vi "CLK机柜开关切换.vi"(6 "OUT":u16, 7 "IN":u16, 8 "error in":errorcluster caption="error constant", 11 "CLK":refnum<k5>) -> (0 "error out":errorcluster caption="error constant", 2 "ask":string)   [LabVIEW 2015]
uses:
  server/Global/SeverGlobal.vi
panel:
  out "Isfailed":bool
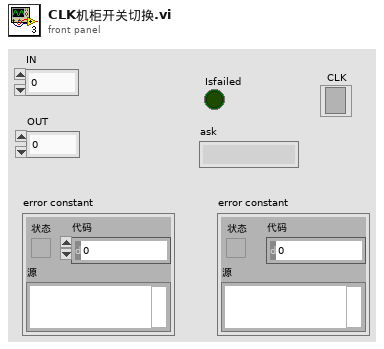
[diagram p1: front panel]
types:
  T1 = enum16{"Standard", "Buffered", "CRLF", "Immediate"}
  T2 = cluster{"IP_A":string, "PORT_A":i32, "IP_B":string, "PORT_B":i32, "IP_CLK":string, "PORT_CLK":i32, "IP_SWITCH":string, "PORT_SWITCH":i32}
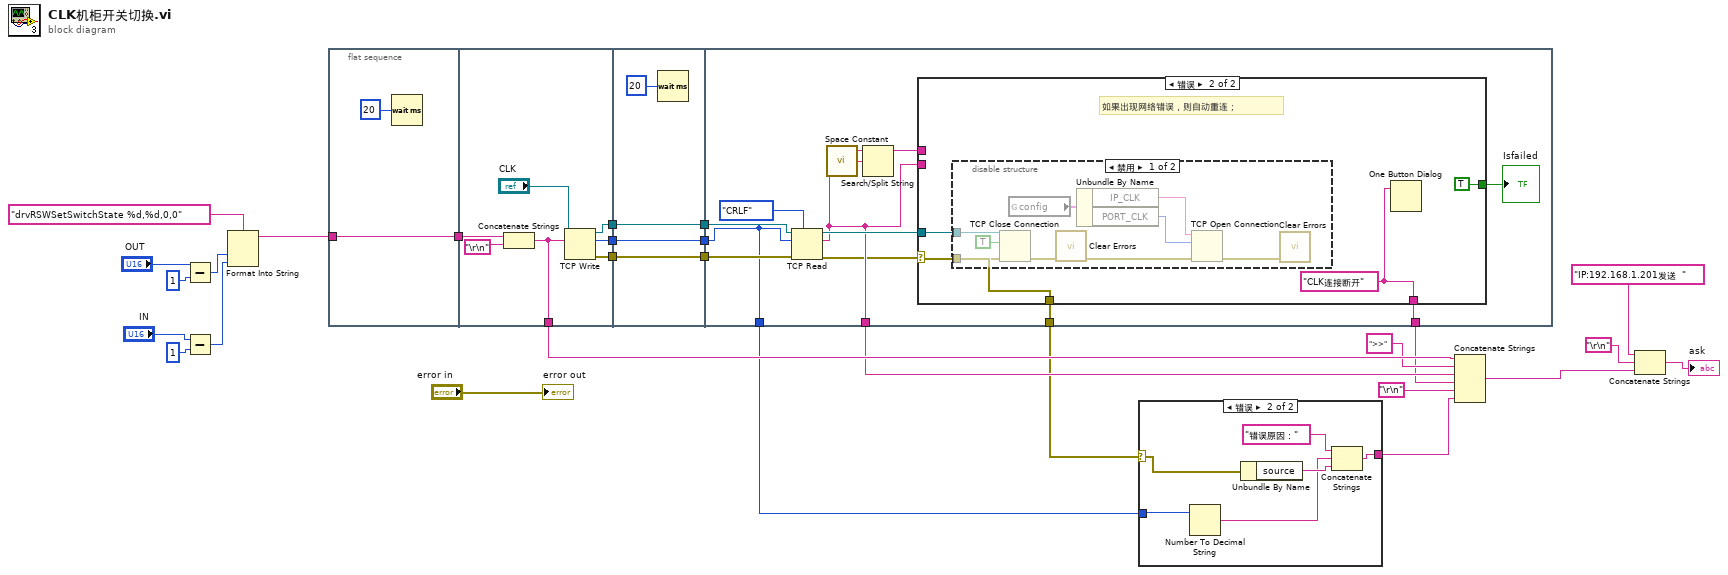
[diagram p0: block diagram]
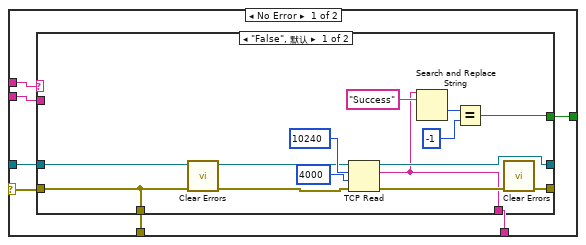
[diagram p3: hidden frame]
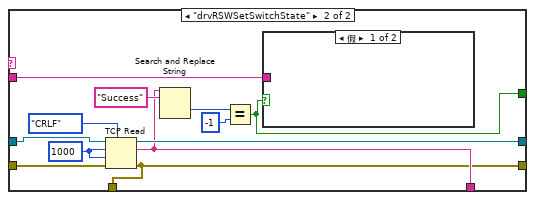
[diagram p4: hidden frame]
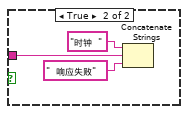
[diagram p5: hidden frame]
diagram:
  n1 = Subtract(x="OUT", y=1) -> (x-y=w19:i32)
  n2 = Subtract(x="IN", y=1) -> (x-y=w17:i32)
  n3 = Format Into String(format string="drvRSWSetSwitchState %d,%d,0,0" ("格式字符串"), w19, w17) -> (resulting string=w16:string)  [unwired: 2 in, 1 out]
  n4 = flat-sequence {
    tunnel: w16 -> [w30]
    tunnel: [w30] -> w28
    tunnel: [w35] -> w27
    tunnel: [w34] -> w26
    tunnel: [w33] -> w25
    tunnel: [w32] -> w9
    tunnel: w28 -> [w36]
    tunnel: [w40] -> w24
    tunnel: w27 -> [w40]
    tunnel: [w39] -> w23
    tunnel: w26 -> [w39]
    tunnel: [w38] -> w22
    tunnel: w25 -> [w38]
    tunnel: w24 -> [w49]
    tunnel: w23 -> [w42]
    tunnel: w22 -> [w48]
    tunnel: [w46] -> w7
    tunnel: [w45] -> w6
    tunnel: [w44] -> w4
    tunnel: [w42] -> w1
    frame #0 {
      n5 = Wait (ms)(milliseconds to wait=u32 20 ("delay")) -> ()  [unwired: 1 out]
    }
    frame #1 {
      n6 = Concatenate Strings(w36, "\r\n") -> (w32:string)
      n7 = TCP Write(connection ID="CLK", data in=w32) -> (connection ID out=w35:refnum<k5>, bytes written=w34:i32, error out=w33:errorcluster)  [unwired: 2 in]
    }
    frame #2 {
      n8 = Wait (ms)(milliseconds to wait=u32 20 ("delay")) -> ()  [unwired: 1 out]
    }
    frame #3 {
      n9 = TCP Read(connection ID=w49, bytes to read=w42, error in (no error)=w48, 7:T1."CRLF" ("mode (standard)")) -> (connection ID out=w50:refnum<k5>, data out=w46:string, error out=w43:errorcluster)  [unwired: 1 in]
      n10 = call <vilib>:"Space Constant.vi"() -> ("String"=w53:string)
      n11 = Search/Split String(string=w46, search string/char (-)=w53) -> (substring before match=w51:string)  [unwired: 1 in, 2 out]
      n12 = case shown="错误" w43 {
        selector: w43 -> [w54 w90]
        tunnel: w51 -> [w60 _]
        tunnel: w50 -> [w59 w92]
        tunnel: [w58 TRUE] -> w47
        tunnel: w46 -> [w57 _]
        tunnel: [w56 w89] -> w45
        tunnel: [w55 w90] -> w44
        frame No Error {
          n13 = case shown="\"False\", 默认" w60 {
            tunnel: [w69 w84] -> _
            tunnel: [w68 w74] -> _
            tunnel: w59 -> [w70 w83]
            tunnel: w54 -> [w61 w82]
            tunnel: w57 -> [_ w77]
            tunnel: [w63 w76] -> w58
            tunnel: [w64 w75] -> w56
            tunnel: [w61 w74] -> w55
            frame "False", Default {
              n14 = call <vilib>:"Clear Errors.vi"("error in (no error)"=w61) -> ("error out"=w62:errorcluster)  [unwired: 5 in, 1 out]
              n15 = TCP Read(connection ID=w70, bytes to read=10240, error in (no error)=w62, 9:4000 ("timeout ms (25000)")) -> (connection ID out=w69:refnum<k5>, data out=w64:string, error out=w72:errorcluster)  [unwired: 1 in]
              n16 = Search and Replace String(input string=w64, search string="Success") -> (offset past replacement=w65:i32)  [unwired: 6 in, 3 out]
              n17 = Equal?(x=w65, y=-1) -> (x = y?=w63:bool)
              n18 = call <vilib>:"Clear Errors.vi"("error in (no error)"=w72) -> ("error out"=w68:errorcluster)  [unwired: 5 in, 1 out]
            }
            frame "drvRSWSetSwitchState" {
              w81 = 1000 ("timeout ms (25000)")
              n19 = TCP Read(connection ID=w83, bytes to read=w81, error in (no error)=w82, 7:T1."CRLF" ("mode (standard)"), 9:w81) -> (connection ID out=w84:refnum<k5>, data out=w75:string, error out=w74:errorcluster)
              n20 = Search and Replace String(input string=w75, search string="Success") -> (offset past replacement=w79:i32)  [unwired: 6 in, 3 out]
              n21 = Equal?(x=w79, y=-1) -> (x = y?=w76:bool)
              n22 = case shown="假" w76 {
                tunnel: w77 -> [_ w88]
                frame False {
                }
                frame True {
                  n23 = Concatenate Strings("时钟  " ("message"), w88, "  响应失败" ("message")) -> ()  [unwired: 1 out]
                }
              }
            }
          }
        }
        frame Error {
          w89 = "CLK连接断开" ("字符串")
          # "如果出现网络错误，则自动重连；"
          n24 = disable-structure shown="禁用" {
            disable-tunnel: w92 -> [w95 _]
            disable-tunnel: w90 -> [w94 _]
            frame Disabled {
              n25 = TCP Close Connection(connection ID=w95, abort (F)=TRUE ("中止(F)"), error in (no error)=w94) -> (error out=w96:errorcluster)  [unwired: 1 out]
              n26 = global read "SeverGlobal.vi" "config"() -> (w98:T2)
              n27 = call <vilib>:"Clear Errors.vi"("error in (no error)"=w96) -> ("error out"=w97:errorcluster)  [unwired: 5 in, 1 out]
              n28 = Unbundle By Name(w98) -> ("IP_CLK"=w99:string, "PORT_CLK"=w100:i32)
              n29 = TCP Open Connection(address=w99, remote port or service name=w100, error in (no error)=w97) -> (error out=w101:errorcluster)  [unwired: 2 in, 1 out]
              n30 = call <vilib>:"Clear Errors.vi"("error in (no error)"=w101) -> ()  [unwired: 5 in, 2 out]
            }
            frame Enabled {
            }
          }
          n31 = One Button Dialog(message=w89) -> ()  [unwired: 1 in, 1 out]
        }
      }
      "Isfailed" <- w47
    }
  }
  n32 = case shown="错误" w4 {
    selector: w4 -> [_ w107]
    tunnel: [_ w105] -> w2
    tunnel: w1 -> [_ w103]
    frame No Error {
    }
    frame Error {
      n33 = Number To Decimal String(number=w103) -> (decimal integer string=w102:string)  [unwired: 1 in]
      n34 = Unbundle By Name(w107) -> ("source"=w104:string)
      n35 = Concatenate Strings("错误原因：", w102, w104) -> (w105:string)
    }
  }
  n36 = Concatenate Strings(w9, ">>" ("字符串"), w7, w6, "\r\n", w2) -> (w5:string)
  n37 = Concatenate Strings("IP:192.168.1.201发送  " ("delimiter (Tab)"), "\r\n", w5) -> (→"ask":string)
  "error out" <- "error in"
